vi "Measurement UI.vi"() -> ()   [LabVIEW 2021, in "adc_acMultiChannelMeasurementUI.lvlib"]
uses:
  adc_acMultiChannelMeasurementUI.lvlib
panel:
  in  "PlotLegends":T1(array[cluster])
  in  "Waveform Result":string(combo)="Frequency Domain"
  in  "PlotLegend":bool
  out "TimeDomainGraph":waveform(dbl)[](graph) caption="AC"
  out "FreqDomainGraph":T2(graph) caption="AC"
  out "MeasTable":string[][](table)
  in  "Digital capture samples":u32 caption="NUMBER OF SAMPLES"
  in  "Digital capture sample rate":dbl=800000.0 caption="SAMPLE RATE" format="%#_6pS/s"
  in  "Digital capture resource name":string(combo) caption="RESOURCE NAME"
  in  "Amplitude":dbl=-1.0 caption="AMPLITUDE" format="%#_6pdB"
  in  "Frequency":dbl=1000.0 caption="FREQUENCY" format="%#_6pHz"
  in  "Full scale range":dbl caption="FULL SCALE RANGE" format="%#_6pV"
  in  "Number of channels":u32=1 caption="NUMBER OF CHANNELS"
  out "Time domain size":i32
  out "Spectrum size":i32
  out "ENOBs":dbl[](array[numeric])
  out "SFDRs":dbl[](array[numeric])
  out "SINADs":dbl[](array[numeric])
  out "THDs":dbl[](array[numeric])
  out "SNRs":dbl[](array[numeric])
  out "Calculated amplitudes":dbl[](array[numeric])
  out "Calculated frequencies":dbl[](array[numeric])
  out "Channel names":string[](array[string])
  in  "Analog source resource names":string[](array[string])
  in  "Analog source input channels":i32[](array[numeric]) min=0 max=100 step=1
  out "Time domain":dbl[](array[numeric])
  out "dt":dbl
  out "t0":dbl
  out "Spectrum":dbl[](array[numeric])
  out "df":dbl
  out "f0":dbl
  in  "Channel parameters":T3(array[cluster]) caption="CHANNEL PARAMETERS"
  out "Digital capture":string="Digital capture"
  out "Analog source":string="Analog source"
  in  "MeasSettingsOptions":i32(listbox)
  in  "MeasSettings":bool
  out "ADCparameters":string="ADC parameters"
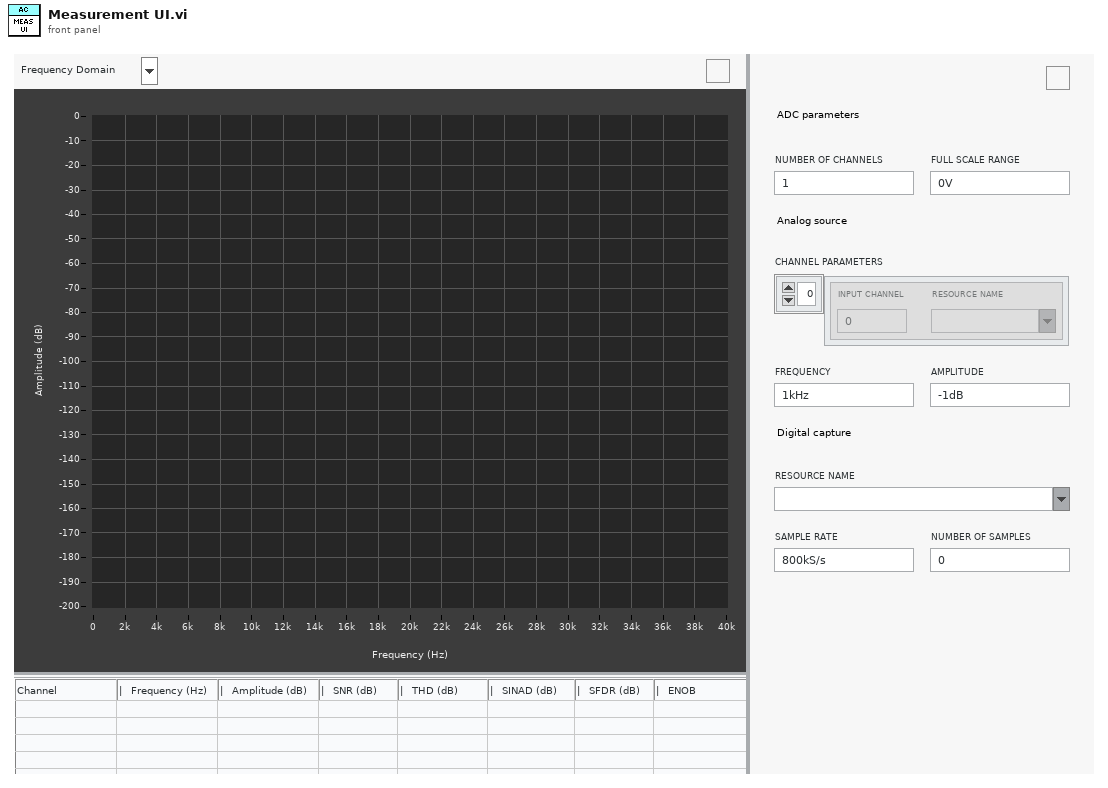
[diagram p1: front panel]
types:
  T1 = cluster{"Color":u32, "Name":string, "Visible":bool}[]
  T2 = cluster{"f0 2":dbl, "df 2":dbl, "Spectrum 2":dbl[]}[]
  T3 = cluster{"Input channel":i32, "Resource name":string}[]
  T4 = enum16{"open", "replace", "create", "open or create", "replace or create", "replace or create with confirmation"}
  T5 = cluster{"Input channel":i32, "Resource name":string}
  T6 = cluster{"Color":u32, "Name":string, "Visible":bool}
  T7 = typedef "LVPoint32TypeDef.ctl" = cluster{"Horizontal":i32, "Vertical":i32}
  T8 = typedef "LVBoundsTypeDef.ctl" = cluster{"Width":u32, "Height":u32}
  T9 = typedef "LVPositionTypeDef.ctl" = cluster{"Left":i32, "Top":i32}
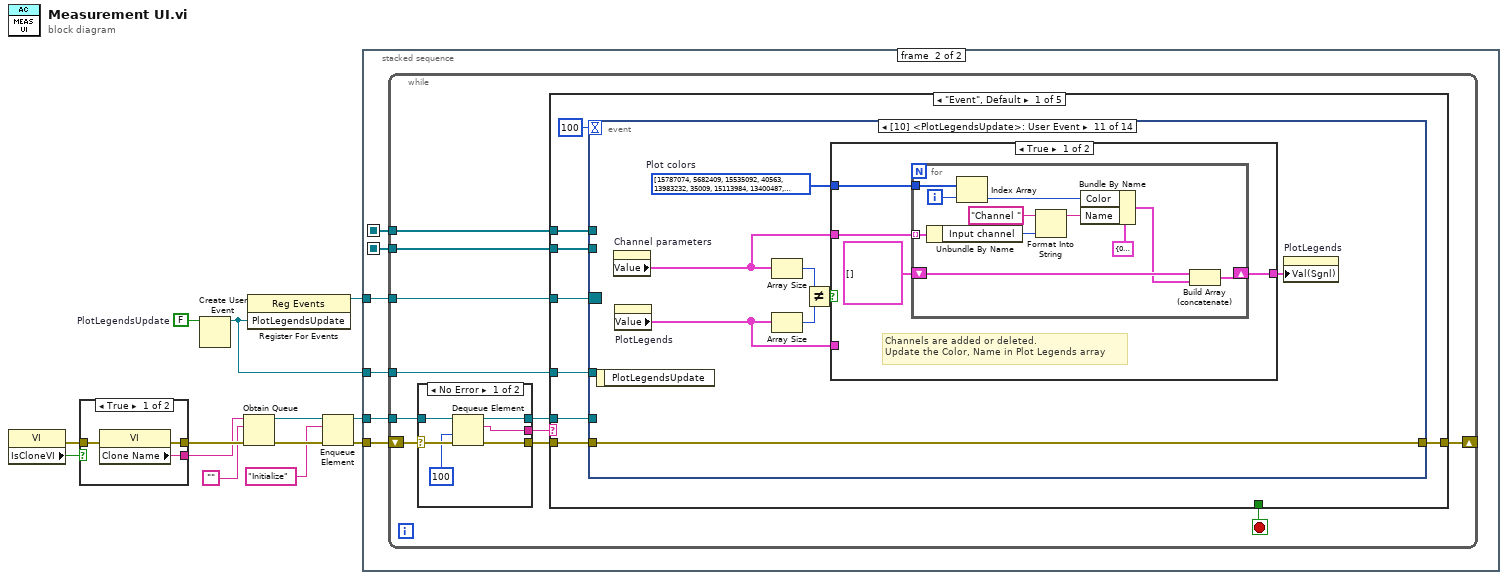
[diagram p0: block diagram]
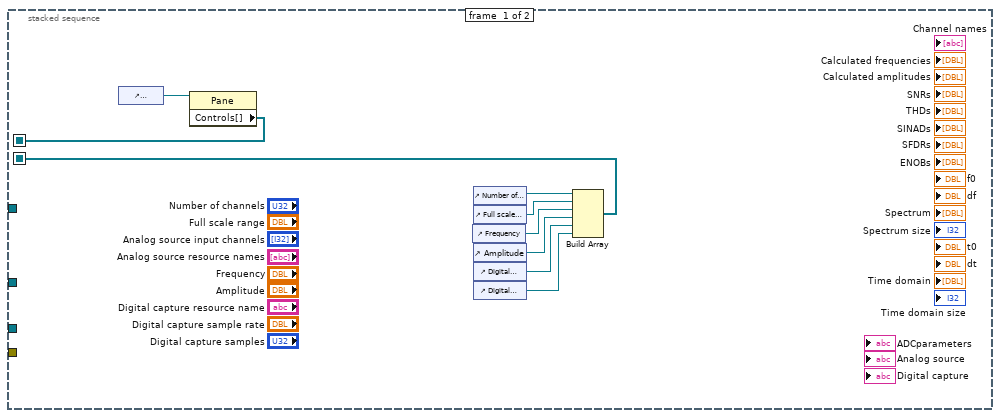
[diagram p2: hidden frame]
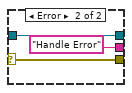
[diagram p3: hidden frame]
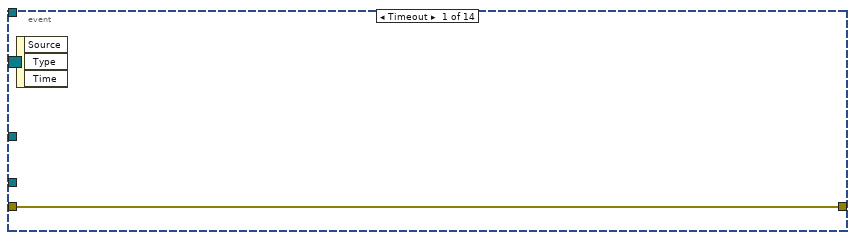
[diagram p4: hidden frame]
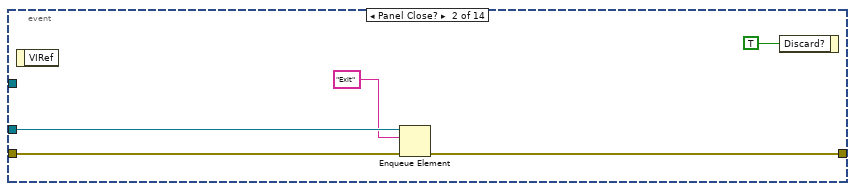
[diagram p5: hidden frame]
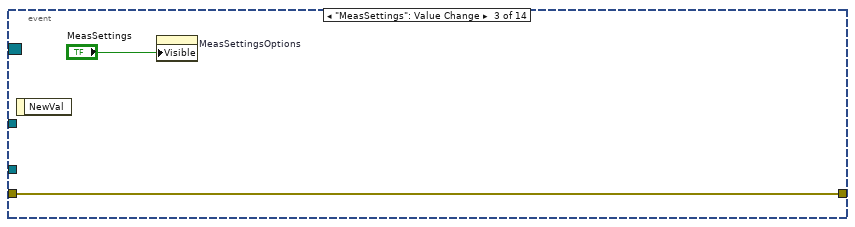
[diagram p6: hidden frame]
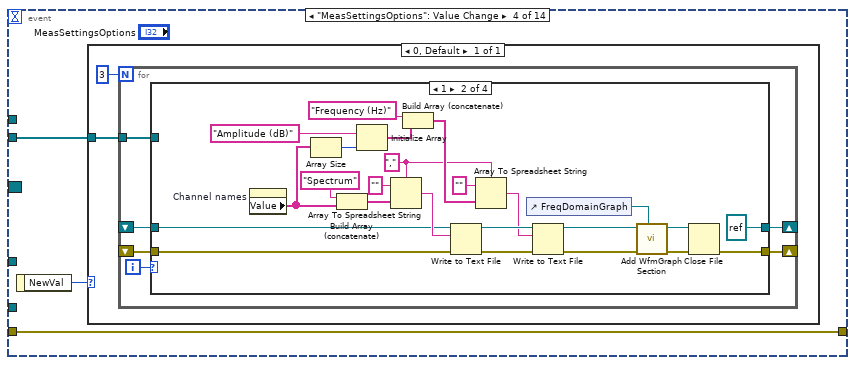
[diagram p7: hidden frame]
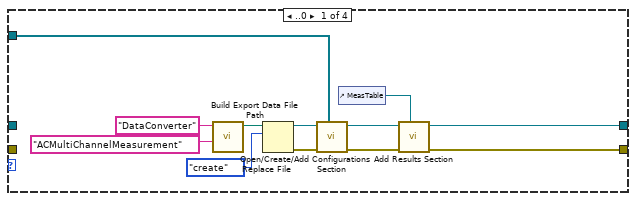
[diagram p8: hidden frame]
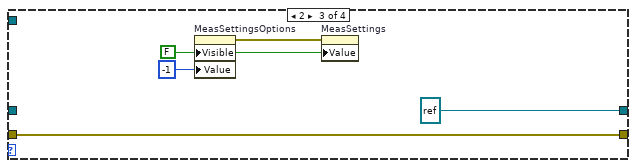
[diagram p9: hidden frame]
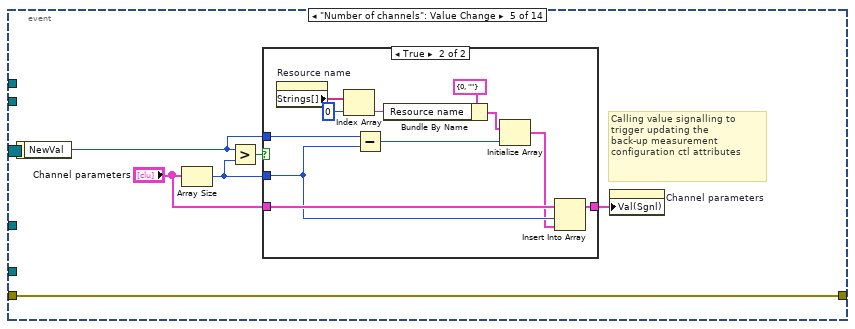
[diagram p11: hidden frame]
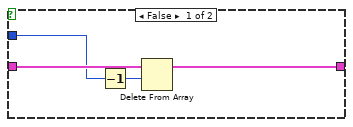
[diagram p12: hidden frame]
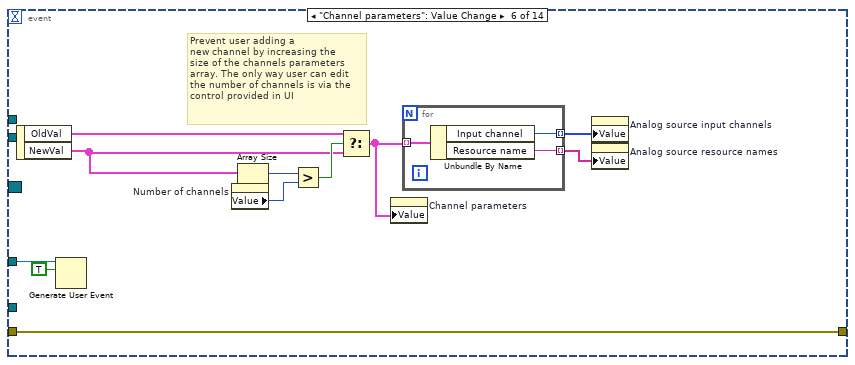
[diagram p13: hidden frame]
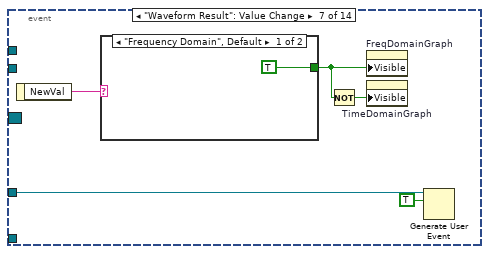
[diagram p14: hidden frame]
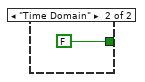
[diagram p15: hidden frame]
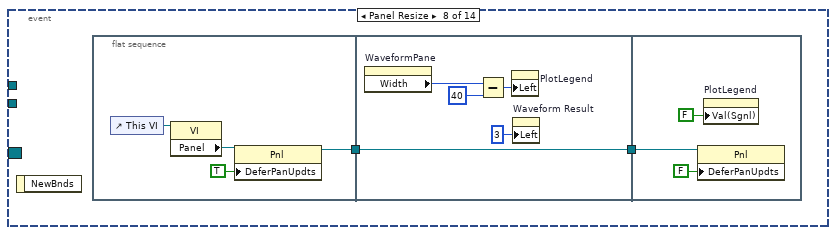
[diagram p16: hidden frame]
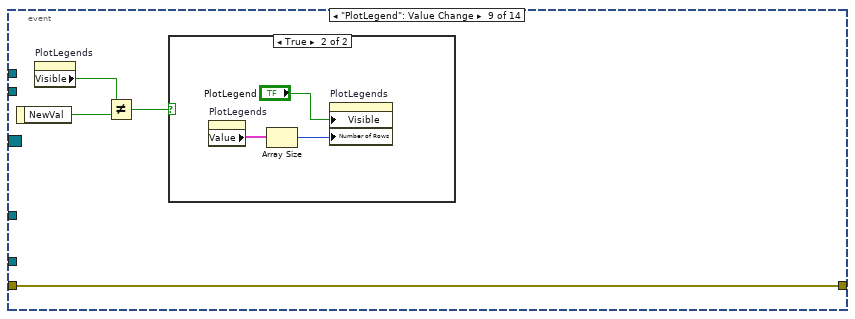
[diagram p17: hidden frame]
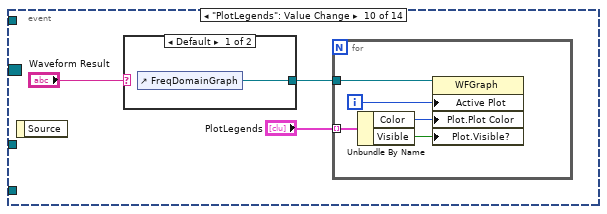
[diagram p19: hidden frame]
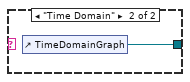
[diagram p20: hidden frame]
diagram:
  w3 = FALSE  # PlotLegendsUpdate
  n1 = property class="VI"() -> (error out=w4:errorcluster, "IsCloneVI"=w5:bool)  [unwired: 2 in, 1 out]
  n2 = case shown="True" w5 {
    tunnel: [w16 w19] -> w13
    tunnel: [w15 w18] -> w12
    tunnel: w4 -> [w14 w17]
    frame True {
      n3 = property class="VI"(error in=w14) -> (error out=w16:errorcluster, "Clone Name"=w15:string)  [unwired: 1 in, 1 out]
    }
    frame False {
      n4 = property class="VI"(error in=w17) -> (error out=w19:errorcluster, "Name"=w18:string)  [unwired: 1 in, 1 out]
    }
  }
  n5 = Create User Event(user event datatype=w3) -> (user event=w1:refnum<user-event>)  [unwired: 1 in, 1 out]
  n6 = Obtain Queue(name (unnamed)=w12, element data type="", error in (no error)=w13) -> (queue out=w9:refnum<queue>, error out=w11:errorcluster)  [unwired: 2 in, 1 out]
  n7 = register-events(w1) -> (reference out=w2:refnum<event-registration>)  [unwired: 2 in, 1 out]
  n8 = Enqueue Element(queue=w9, element="Initialize", error in (no error)=w11) -> (queue out=w8:refnum<queue>, error out=w10:errorcluster)  [unwired: 1 in, 1 out]
  n9 = stacked-sequence {
    seq-local: [w27 _] -> [_ w32]
    seq-local: [w22 _] -> [_ w29]
    tunnel: w10 -> [_ w34]
    tunnel: w8 -> [_ w33]
    tunnel: w2 -> [_ w31]
    tunnel: w1 -> [_ w30]
    frame #0 {
      n10 = control-ref of="WaveformPane"() -> (w21:refnum<vi>)
      n11 = property class="Pane"(reference=w21) -> ("Controls[]"=w22:refnum<vi>[])  [unwired: 1 in, 2 out]
      n12 = control-ref of="Frequency"() -> (w20:refnum<vi>)
      n13 = control-ref of="Number of channels"() -> (w28:refnum<vi>)
      n14 = control-ref of="Full scale range"() -> (w23:refnum<vi>)
      n15 = control-ref of="Amplitude"() -> (w26:refnum<vi>)
      n16 = control-ref of="Digital capture sample rate"() -> (w25:refnum<vi>)
      n17 = control-ref of="Digital capture samples"() -> (w24:refnum<vi>)
      n18 = Build Array(w28, w23, w20, w26, w25, w24) -> (w27:refnum<vi>[])
    }
    frame #1 {
      n19 = while {
        shift-right: [w40] -> _
        shift-left: w34 -> [w45]
        tunnel: w33 -> [w43]
        tunnel: w32 -> [w38]
        tunnel: w31 -> [w37]
        tunnel: w30 -> [w36]
        tunnel: w29 -> [w35]
        stop <- w39 stop-if-true
        n20 = case shown="No Error" w45 {
          selector: w45 -> [w51 w54]
          tunnel: [w50 w54] -> w44
          tunnel: w43 -> [w49 w53]
          tunnel: [w48 w53] -> w42
          tunnel: [w47 "Handle Error"] -> w41
          frame No Error {
            n21 = Dequeue Element(queue=w49, timeout in ms (-1)=100, error in (no error)=w51) -> (queue out=w48:refnum<queue>, element=w47:string, error out=w50:errorcluster)  [unwired: 1 out]
          }
          frame Error {
          }
        }
        n22 = case shown="\"Event\", Default" w41 {
          tunnel: w44 -> [w61 w257 w302 w330 w331]
          tunnel: w42 -> [w59 _ _ w328 _]
          tunnel: [w62 w257 w302 w325 w331] -> w40
          tunnel: [_ _ _ TRUE _] -> w39
          tunnel: w38 -> [w58 _ _ _ _]
          tunnel: w37 -> [w57 _ _ _ _]
          tunnel: w36 -> [w56 _ _ _ _]
          tunnel: w35 -> [w55 _ _ _ _]
          frame "Event", Default {
            n23 = event shown="[10] <PlotLegendsUpdate>: User Event" {
              selector: w57 -> [_ _ _ _ _ _ _ _ _ _ _ _ _ _]
              dyn-events: _ -> [_ _ _ _ _ _ _ _ _ _ _ _ _ _]
              timeout: 100 -> [_ _ _ _ _ _ _ _ _ _ _ _ _ _]
              tunnel: [w63 w66 w70 w72 w130 w156 _ _ w184 _ w205 w236 _ _] -> w62
              tunnel: w61 -> [w63 w67 w70 w72 w130 w156 _ _ w184 _ w205 w236 _ _]
              tunnel: w59 -> [_ w65 _ _ _ _ _ _ _ _ _ _ _ _]
              tunnel: w58 -> [_ _ _ w71 _ _ _ _ _ _ _ _ _ _]
              tunnel: w56 -> [_ _ _ _ _ w147 w161 _ _ _ _ _ _ _]
              tunnel: w55 -> [_ _ _ _ _ _ _ _ _ _ _ _ _ w242]
              event Timeout {
                n24 = event-data() -> ()  [unwired: 1 in, 3 out]
              }
              event Panel Close? {
                n25 = event-data() -> ()  [unwired: 1 in, 1 out]
                n26 = Enqueue Element(queue=w65, element="Exit", error in (no error)=w67) -> (error out=w66:errorcluster)  [unwired: 1 in, 2 out]
                n27 = event-data("Discard?"=TRUE) -> ()  [unwired: 1 in, 1 out]
              }
              event "MeasSettings": Value Change {
                n28 = event-data() -> ()  [unwired: 1 in, 1 out]
                n29 = property on="MeasSettingsOptions" class="LstBox (strict)"("Visible"="MeasSettings") -> ()  [unwired: 2 in, 2 out]
              }
              event "MeasSettingsOptions": Value Change {
                n30 = event-data() -> ("NewVal"=w73:i32)  [unwired: 1 in]
                n31 = case shown="0, Default" w73 {
                  tunnel: w71 -> [w74]
                  frame 0, Default {
                    n32 = for {
                      N: 3 -> [_]
                      shift-right: [w80] -> _
                      shift-left: _ -> [w79]
                      shift-right: [w78] -> _
                      shift-left: _ -> [w77]
                      tunnel: w74 -> [w76]
                      i -> [w81]
                      n33 = case shown="1" w81 {
                        tunnel: [w83 refnum<file> refnum ("refnum out") refnum<file> refnum ("refnum out") w124] -> w80
                        tunnel: w79 -> [_ w102 _ w124]
                        tunnel: [w82 w95 w121 w123] -> w78
                        tunnel: w77 -> [_ w101 w121 w123]
                        tunnel: w76 -> [w87 _ _ _]
                        frame ..0 {
                          n34 = call "Build Export Data File Path.vi"("Meas name"="ACMultiChannelMeasurement" ("prompt"), "Plugin name"="DataConverter" ("prompt")) -> ("Export data file path"=w90:path)  [unwired: 9 in]
                          n35 = Open/Create/Replace File(file path (use dialog)=w90, operation (0:open)=T4."create") -> (refnum out=w89:refnum<file>, error out=w88:errorcluster)  [unwired: 4 in, 1 out]
                          n36 = call "Add Configurations Section.vi"("Control references"=w87, "error in"=w88, "File refnum in"=w89) -> ("error out"=w85:errorcluster, "File refnum out"=w86:refnum<file>)  [unwired: 7 in]
                          n37 = control-ref of="MeasTable"() -> (w84:refnum<vi>)
                          n38 = call "Add Results Section.vi"("MeasTable"=w84, "error in"=w85, "File refnum in"=w86) -> ("error out"=w82:errorcluster, "File refnum out"=w83:refnum<file>)  [unwired: 7 in]
                        }
                        frame 1 {
                          w109 = "," ("delimiter (Tab)")
                          n39 = property on="Channel names" class="Arr (strict)"() -> ("Value"=w113:string[])  [unwired: 2 in, 2 out]
                          n40 = Array Size(array=w113) -> (size(s)=w112:i32)
                          n41 = Build Array (concatenate)("Spectrum" ("string"), w113) -> (w116:string[])
                          n42 = Initialize Array("Amplitude (dB)" ("element"), w112) -> (w111:string[])
                          n43 = Array To Spreadsheet String(delimiter (Tab)=w109, array=w116, 3:"" ("format string")) -> (spreadsheet string=w114:string)
                          n44 = Build Array (concatenate)("Frequency (Hz)" ("element"), w111) -> (w110:string[])
                          n45 = Write to Text File(file (use dialog)=w102, text=w114, error in=w101) -> (refnum out=w107:refnum<file>, error out=w106:errorcluster)  [unwired: 1 in, 1 out]
                          n46 = Array To Spreadsheet String(delimiter (Tab)=w109, array=w110, 3:"" ("format string")) -> (spreadsheet string=w105:string)
                          n47 = control-ref of="FreqDomainGraph"() -> (w98:refnum<vi>)
                          n48 = Write to Text File(file (use dialog)=w107, text=w105, error in=w106) -> (refnum out=w100:refnum<file>, error out=w99:errorcluster)  [unwired: 1 in, 1 out]
                          n49 = call "Add WfmGraph Section.vi"("Waveform Graph"=w98, "error in"=w99, "File refnum in"=w100) -> ("error out"=w96:errorcluster, "File refnum out"=w97:refnum<file>)  [unwired: 7 in]
                          n50 = Close File(refnum=w97, error in=w96) -> (error out=w95:errorcluster)  [unwired: 1 out]
                        }
                        frame 2 {
                          w119 = FALSE ("Visible")
                          n51 = property on="MeasSettingsOptions" class="LstBox (strict)"("Visible"=w119, "Value"=-1 ("MeasSettingsOptions")) -> (error out=w120:errorcluster)  [unwired: 2 in, 1 out]
                          n52 = property on="MeasSettings" class="Bool (strict)"(error in=w120, "Value"=w119) -> ()  [unwired: 1 in, 2 out]
                        }
                        frame Default {
                        }
                      }
                    }
                  }
                }
              }
              event "Number of channels": Value Change {
                # "Calling value signalling to trigger updating the\nback-up measurement configuration ctl attributes"
                n53 = event-data() -> ("NewVal"=w129:u32)  [unwired: 1 in]
                n54 = Array Size(array="Channel parameters") -> (size(s)=w126:i32)
                n55 = Greater?(x=w129, y=w126) -> (0:w128:bool)
                n56 = case shown="True" w128 {
                  tunnel: "Channel parameters" -> [w134 w145]
                  tunnel: w126 -> [w131 w143]
                  tunnel: w129 -> [_ w144]
                  tunnel: [w133 w141] -> w125
                  frame False {
                    n57 = Decrement(x=w131) -> (x-1=w132:i32)
                    n58 = Delete From Array(array=w134, length=w132) -> (array with subset deleted=w133:T3)  [unwired: 1 in, 1 out]
                  }
                  frame True {
                    n59 = property on="Resource name" class="CmbBox"() -> ("Strings[]"=w139:string[])  [unwired: 2 in, 2 out]
                    n60 = Index Array(array=w139, index=0) -> (element=w137:string)
                    n61 = Subtract(x=w144, y=w143) -> (x-y=w142:u32)
                    n62 = Bundle By Name(cluster=T5 {"Input channel"=0, "Resource name"=""} ("Cluster"), "Resource name"=w137) -> (w135:T5)
                    n63 = Initialize Array(w135, w142) -> (w140:T3)
                    n64 = Insert Into Array(array=w145, index=w143, new element=w140) -> (w141:T3)
                  }
                }
                n65 = property on="Channel parameters" class="Arr (strict)"("Val(Sgnl)"=w125) -> ()  [unwired: 2 in, 2 out]
              }
              event "Channel parameters": Value Change {
                # "Prevent user adding a \nnew channel by increasing the\nsize of the channels parameters\narray. The only way user can edit\nthe number of channels is via the\ncontrol provided in UI"
                n66 = event-data() -> ("OldVal"=w152:T3, "NewVal"=w151:T3)  [unwired: 1 in]
                n67 = Generate User Event(user event=w147, event data cluster=TRUE ("event data")) -> ()  [unwired: 2 in, 2 out]
                n68 = property on="Number of channels" class="DigNum (strict)"() -> ("Value"=w154:u32)  [unwired: 2 in, 2 out]
                n69 = Array Size(array=w151) -> (size(s)=w155:i32)
                n70 = Greater?(x=w155, y=w154) -> (0:w153:bool)
                n71 = Select(t=w152, s=w153, f=w151) -> (s? t:f=w150:T3)
                n72 = property on="Channel parameters" class="Arr (strict)"("Value"=w150) -> ()  [unwired: 2 in, 2 out]
                n73 = for {
                  tunnel: w150 -> [w159] mode=indexing
                  tunnel: [w158] -> w149 mode=indexing
                  tunnel: [w157] -> w148 mode=indexing
                  n74 = Unbundle By Name(w159) -> ("Input channel"=w158:i32, "Resource name"=w157:string)
                }
                n75 = property on="Analog source input channels" class="Arr (strict)"("Value"=w149) -> ()  [unwired: 2 in, 2 out]
                n76 = property on="Analog source resource names" class="Arr (strict)"("Value"=w148) -> ()  [unwired: 2 in, 2 out]
              }
              event "Waveform Result": Value Change {
                n77 = event-data() -> ("NewVal"=w164:string)  [unwired: 1 in]
                n78 = case shown="\"Frequency Domain\", Default" w164 {
                  tunnel: [TRUE FALSE] -> w163
                  frame "Frequency Domain", Default {
                  }
                  frame "Time Domain" {
                  }
                }
                n79 = Not(x=w163) -> (.not. x?=w162:bool)
                n80 = property on="FreqDomainGraph" class="WFGraph (strict)"("Visible"=w163) -> ()  [unwired: 2 in, 2 out]
                n81 = property on="TimeDomainGraph" class="WFGraph (strict)"("Visible"=w162) -> ()  [unwired: 2 in, 2 out]
                n82 = Generate User Event(user event=w161, event data cluster=TRUE ("event data")) -> ()  [unwired: 2 in, 2 out]
              }
              event Panel Resize {
                n83 = event-data() -> ()  [unwired: 1 in, 1 out]
                n84 = flat-sequence {
                  tunnel: [w169] -> w167
                  tunnel: [w173] -> w168
                  tunnel: w167 -> [w173]
                  tunnel: w168 -> [w179]
                  frame #0 {
                    n85 = control-ref of="This VI"() -> (w172:refnum<vi>)
                    n86 = property class="VI"(reference=w172) -> ("Panel"=w171:refnum<vi>)  [unwired: 1 in, 2 out]
                    n87 = property class="Pnl"(reference=w171, "DeferPanUpdts"=TRUE ("Defer Panel Updates")) -> (reference out=w169:refnum<vi>)  [unwired: 1 in, 1 out]
                  }
                  frame #1 {
                    n88 = property on="WaveformPane" class="Pane"() -> ("Width"=w176:u32)  [unwired: 2 in, 2 out]
                    n89 = Subtract(x=w176, y=u32 40) -> (x-y=w177:u32)
                    n90 = property on="PlotLegend" class="Bool (strict)"("Left"=w177) -> ()  [unwired: 2 in, 2 out]
                    n91 = property on="Waveform Result" class="CmbBox"("Left"=3 ("Position:Left")) -> ()  [unwired: 2 in, 2 out]
                  }
                  frame #2 {
                    n92 = property class="Pnl"(reference=w179, "DeferPanUpdts"=FALSE ("Defer Panel Updates")) -> ()  [unwired: 1 in, 2 out]
                    n93 = property on="PlotLegend" class="Bool (strict)"("Val(Sgnl)"=FALSE ("Visible")) -> ()  [unwired: 2 in, 2 out]
                  }
                }
              }
              event "PlotLegend": Value Change {
                n94 = event-data() -> ("NewVal"=w183:bool)  [unwired: 1 in]
                n95 = property on="PlotLegends" class="Arr (strict)"() -> ("Visible"=w182:bool)  [unwired: 2 in, 2 out]
                n96 = Not Equal?(x=w182, y=w183) -> (x != y?=w181:bool)
                n97 = case shown="True" w181 {
                  frame False {
                  }
                  frame True {
                    n98 = property on="PlotLegends" class="Arr (strict)"() -> ("Value"=w187:T1)  [unwired: 2 in, 2 out]
                    n99 = Array Size(array=w187) -> (size(s)=w186:i32)
                    n100 = property on="PlotLegends" class="Arr (strict)"("Visible"="PlotLegend", "Number of Rows"=w186) -> ()  [unwired: 2 in, 2 out]
                  }
                }
              }
              event "PlotLegends": Value Change {
                n101 = event-data() -> ()  [unwired: 1 in, 1 out]
                n102 = case shown="Default" "Waveform Result" {
                  tunnel: [w191 w192] -> w189
                  frame Default {
                    n103 = control-ref of="FreqDomainGraph"() -> (w191:refnum<vi>)
                  }
                  frame "Time Domain" {
                    n104 = control-ref of="TimeDomainGraph"() -> (w192:refnum<vi>)
                  }
                }
                n105 = for {
                  tunnel: "PlotLegends" -> [w195] mode=indexing
                  tunnel: w189 -> [w197]
                  i -> [w196]
                  n106 = Unbundle By Name(w195) -> ("Color"=w194:u32, "Visible"=w193:bool)
                  n107 = property class="WFGraph"(reference=w197, "Active Plot"=w196, "Plot.Plot Color"=w194, "Plot.Visible?"=w193) -> ()  [unwired: 1 in, 2 out]
                }
              }
              event User Event {
                w198 = u32[] [15787074, 5682409, 15535092, 40563, 13983232, 35009, 15113984, 13400487, 15993633, 10221451, 8148942, 15869817, 32914, 10196480, 6271923, 16355671]  # Plot colors
                n108 = event-data() -> ()  [unwired: 1 in, 1 out]
                n109 = property on="Channel parameters" class="Arr (strict)"() -> ("Value"=w201:T3)  [unwired: 2 in, 2 out]
                n110 = property on="PlotLegends" class="Arr (strict)"() -> ("Value"=w200:T1)  [unwired: 2 in, 2 out]
                n111 = Array Size(array=w201) -> (size(s)=w203:i32)
                n112 = Array Size(array=w200) -> (size(s)=w202:i32)
                n113 = Not Equal?(x=w203, y=w202) -> (x != y?=w204:bool)
                n114 = case shown="True" w204 {
                  tunnel: w201 -> [w209 w223]
                  tunnel: w198 -> [w208 _]
                  tunnel: [w206 w222] -> w199
                  tunnel: w200 -> [_ w221]
                  frame True {
                    # "Channels are added or deleted. \nUpdate the Color, Name in Plot Legends array"
                    n115 = for {
                      shift-right: [w210] -> w206
                      shift-left: T1 [] -> [w220]
                      tunnel: w209 -> [w215] mode=indexing
                      tunnel: w208 -> [w214]
                      i -> [w213]
                      n116 = Unbundle By Name(w215) -> ("Input channel"=w217:i32)
                      n117 = Index Array(array=w214, index=w213) -> (element=w212:u32)
                      n118 = Format Into String(initial string="Channel ", w217) -> (resulting string=w216:string)  [unwired: 2 in, 1 out]
                      n119 = Bundle By Name(cluster=T6 {"Color"=0, "Name"="", "Visible"=TRUE} ("new element/subarray"), "Color"=w212, "Name"=w216) -> (w211:T6)
                      n120 = Build Array (concatenate)(w220, w211) -> (w210:T1)
                    }
                  }
                  frame False {
                    # "Channel number is updated in UI\nUpdate the Channel name in Plot Legends array"
                    n121 = for {
                      shift-right: [w228] -> w222
                      shift-left: w221 -> [w226]
                      tunnel: w223 -> [w229] mode=indexing
                      i -> [w224]
                      n122 = Unbundle By Name(w229) -> ("Input channel"=w231:i32)
                      n123 = Index Array(array=w226, index=w224) -> (element=w225:T6)
                      n124 = Format Into String(initial string="Channel ", w231) -> (resulting string=w230:string)  [unwired: 2 in, 1 out]
                      n125 = Bundle By Name(cluster=w225, "Name"=w230) -> (w227:T6)
                      n126 = Replace Array Subset(array=w226, new element=w227, index=w224) -> (w228:T1)
                    }
                  }
                }
                n127 = property on="PlotLegends" class="Arr (strict)"("Val(Sgnl)"=w199) -> ()  [unwired: 2 in, 2 out]
              }
              event Mouse Down {
                w234 = FALSE ("Visible")
                n128 = event-data() -> ()  [unwired: 1 in, 1 out]
                n129 = property on="MeasSettingsOptions" class="LstBox (strict)"("Visible"=w234, "Value"=-1 ("MeasSettingsOptions")) -> (error out=w235:errorcluster)  [unwired: 2 in, 1 out]
                n130 = property on="PlotLegend" class="Bool (strict)"("Val(Sgnl)"=FALSE ("Visible")) -> ()  [unwired: 2 in, 2 out]
                n131 = property on="MeasSettings" class="Bool (strict)"(error in=w235, "Value"=w234) -> ()  [unwired: 1 in, 2 out]
              }
              event Mouse Down {
                n132 = event-data() -> ()  [unwired: 1 in, 1 out]
                n133 = property on="PlotLegend" class="Bool (strict)"("Val(Sgnl)"=FALSE ("Visible")) -> ()  [unwired: 2 in, 2 out]
              }
              event Mouse Down? {
                n134 = event-data() -> ("Coords"=w241:T7)  [unwired: 1 in]
                n135 = for {
                  tunnel: w242 -> [w256] mode=indexing
                  tunnel: w241 -> [w255]
                  tunnel: [w246] -> w240
                  stop <- w247 stop-if-true
                  # "Identify the control where Mouse down\nevent happened"
                  n136 = property class="Ctl"(reference=w256) -> ("Label.Text"=w246:string, "Bounds"=w254:T8, "Position"=w251:T9)  [unwired: 1 in, 2 out]
                  n137 = To Long Integer(number=w254) -> (32bit integer=w253:cluster{"Width":i32, "Height":i32})
                  n138 = Add(x=w253, y=w251) -> (x+y=w252:T9)
                  n139 = In Range and Coerce(upper limit=w252, x=w255, lower limit=w251) -> (In Range?=w250:cluster{"Left":bool, "Top":bool})  [unwired: 1 out]
                  n140 = Unbundle By Name(w250) -> ("Left"=w249:bool, "Top"=w248:bool)
                  n141 = And(x=w249, y=w248) -> (x .and. y?=w247:bool)
                }
                n142 = case shown="\"PlotLegend\", \"PlotLegends\"" w240 {
                  tunnel: [TRUE FALSE] -> w239
                  frame "False", Default {
                  }
                  frame "PlotLegend", "PlotLegends" {
                    # "If Mouse is clicked anywhere\nother than the Plot Legends or\nthe Eye Icon, then Hide the\nPlot legends"
                  }
                }
                n143 = case shown="True" w239 {
                  frame False {
                  }
                  frame True {
                    n144 = property on="PlotLegend" class="Bool (strict)"("Val(Sgnl)"=FALSE ("Visible")) -> ()  [unwired: 2 in, 2 out]
                  }
                }
                n145 = event-data() -> ()  [unwired: 2 in, 1 out]
              }
            }
          }
          frame "Initialize" {
            n146 = stacked-sequence {
              frame #0 {
                w268 = string[] ["Export data"] ("Item Names")
                n147 = property on="Channel parameters" class="Arr (strict)"("Value"=T3 [] ("Channel parameters")) -> (error out=w261:errorcluster)  [unwired: 2 in, 1 out]
                n148 = call "Detected DPIs.vi"() -> ("DPI resources"=w260:string[])  [unwired: 10 in, 1 out]
                n149 = call "Detected DSGs.vi"() -> ("AO channels"=w264:string[])  [unwired: 11 in]
                n150 = Index Array(array=w260) -> (element=w259:string)  [unwired: 1 in]
                n151 = Index Array(array=w264) -> (element=w263:string)  [unwired: 1 in]
                n152 = property on="MeasSettingsOptions" class="LstBox (strict)"("Item Names"=w268, "Value"=-1 ("MeasSettingsOptions"), "Visible"=FALSE, "Disabled Items"=i32[] []) -> ()  [unwired: 2 in, 2 out]
                n153 = property on="Resource name" class="CmbBox"(error in=w261, "Strings[]"=w264, "Value"=w263) -> (error out=w258:errorcluster)  [unwired: 1 in, 1 out]
                n154 = for {
                  tunnel: w268 -> [_] mode=indexing
                  i -> [w270]
                  n155 = property on="MeasSettingsOptions" class="LstBox (strict)"("Active Row"=w270, "Cell Height"=30 ("Active Row:Cell Height")) -> ()  [unwired: 2 in, 2 out]
                }
                n156 = property on="Digital capture resource name" class="CmbBox"(error in=w258, "Strings[]"=w260, "Value"=w259) -> ()  [unwired: 1 in, 2 out]
              }
              frame #1 {
                n157 = property on="Number of channels" class="DigNum (strict)"("Val(Sgnl)"=u32 1 ("Value (Signaling)")) -> (error out=w271:errorcluster)  [unwired: 2 in, 1 out]
                n158 = property on="PlotLegend" class="Bool (strict)"(error in=w271, "Val(Sgnl)"=FALSE ("Visible")) -> ()  [unwired: 1 in, 2 out]
              }
            }
          }
          frame "Post UI Update" {
            # "This case will be triggered, after framework updates the User interface with result values."
            n159 = local read "Spectrum size"() -> (w296:i32)
            n160 = local read "Spectrum"() -> (w298:dbl[])
            n161 = local read "Calculated frequencies"() -> (w290:dbl[])
            n162 = local read "Calculated amplitudes"() -> (w289:dbl[])
            n163 = local read "SINADs"() -> (w286:dbl[])
            n164 = Array Size(array=w298) -> (size(s)=w299:i32)
            n165 = local read "ENOBs"() -> (w284:dbl[])
            n166 = local read "SFDRs"() -> (w285:dbl[])
            n167 = local read "THDs"() -> (w287:dbl[])
            n168 = local read "SNRs"() -> (w288:dbl[])
            n169 = local read "df"() -> (w301:dbl)
            n170 = local read "f0"() -> (w300:dbl)
            n171 = Quotient & Remainder(x=w299, y=w296) -> (floor(x/y)=w297:i32)  [unwired: 1 out]
            n172 = for {
              N: w297 -> [_]
              shift-right: [w322] -> _
              shift-left: w298 -> [w323]
              tunnel: w296 -> [w321]
              tunnel: w300 -> [w320]
              tunnel: w301 -> [w319]
              tunnel: [w317] -> w275 mode=indexing
              n173 = Delete From Array(array=w323, length=w321) -> (deleted portion=w318:dbl[], array with subset deleted=w322:dbl[])  [unwired: 1 in]
              n174 = Bundle("f0"=w320, "df"=w319, "Spectrum"=w318) -> (w317:cluster{"f0":dbl, "df":dbl, "Spectrum":dbl[]})  [unwired: 1 in]
            }
            "FreqDomainGraph" <- w275
            n175 = Build Array(w290, w289, w288, w287, w286, w285, w284) -> (w283:dbl[][])
            n176 = for {
              tunnel: w283 -> [w306] mode=indexing
              tunnel: [w305] -> w280 mode=indexing
              tunnel: string[] ["%.3f", "%.3f", "%5.1f", "%5.1f", "%5.1f", "%5.1f", "%5.1f"] -> [w304] mode=indexing
              tunnel: "|   " ("initial string") -> [w303]
              n177 = for {
                tunnel: w306 -> [w310] mode=indexing
                tunnel: [w309] -> w305 mode=indexing
                tunnel: w304 -> [w308]
                tunnel: w303 -> [w307]
                n178 = Format Into String(format string=w308, initial string=w307, w310) -> (resulting string=w309:string)  [unwired: 1 in, 1 out]
              }
            }
            n179 = local read "Time domain size"() -> (w294:i32)
            n180 = local read "Time domain"() -> (w292:dbl[])
            n181 = local read "Channel names"() -> (w279:string[])
            n182 = Array Size(array=w292) -> (size(s)=w291:i32)
            n183 = local read "dt"() -> (w295:dbl)
            n184 = Quotient & Remainder(x=w291, y=w294) -> (floor(x/y)=w293:i32)  [unwired: 1 out]
            n185 = Insert Into Array(array=w280, index (row)=0, new element=w279) -> (w278:string[][])  [unwired: 1 in]
            n186 = for {
              N: w293 -> [_]
              shift-right: [w315] -> _
              shift-left: w292 -> [w316]
              tunnel: w294 -> [w314]
              tunnel: [w312] -> w274 mode=indexing
              tunnel: w295 -> [w311]
              n187 = Delete From Array(array=w316, length=w314) -> (deleted portion=w313:dbl[], array with subset deleted=w315:dbl[])  [unwired: 1 in]
              n188 = Bundle By Name("dt"=w311, "Y"=w313) -> (w312:waveform(dbl))  [unwired: 1 in]
            }
            "TimeDomainGraph" <- w274
            n189 = Transpose 2D Array(2D array=w278) -> (transposed array=→"MeasTable":string[][])
          }
          frame "Exit" {
            # "This case is triggered to close the User Interface from framework"
            n190 = Flush Queue(queue=w328, error in (no error)=w330) -> (queue out=w327:refnum<queue>, error out=w326:errorcluster)  [unwired: 1 out]
            n191 = Release Queue(queue=w327, force destroy? (F)=TRUE, error in (no error)=w326) -> (error out=w325:errorcluster)  [unwired: 2 out]
          }
          frame "Handle Error" {
          }
        }
      }
    }
  }
